vi "Create.vi"(8 "error in (no error)":errorcluster, 11 "DataSocketMessenger in":refnum<class "DataSocketMessenger.lvclass">) -> (0 "error out":errorcluster, 3 "DataSocketMessenger out":refnum<class "DataSocketMessenger.lvclass">)   [LabVIEW 2011, in "Messenging.lvlib" / "DataSocketMessenger.lvclass"]
uses:
  DataSocketMessenger.lvclass
  DataSocketMessenger.lvclass/DataSocketMessenger.ctl
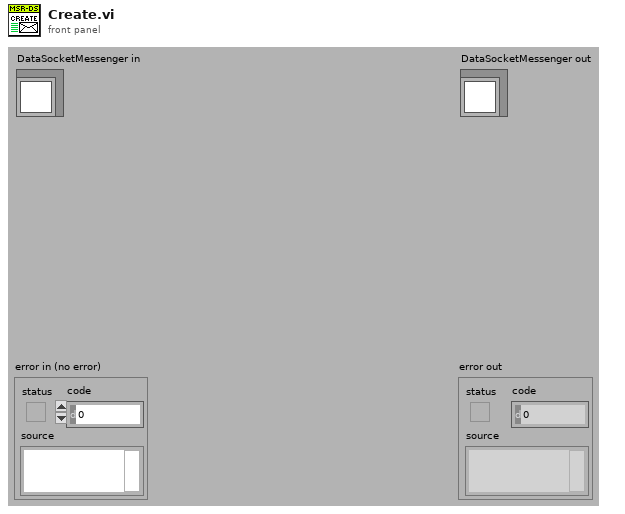
[diagram p1: front panel]
types:
  T1 = enum16{"Read", "Write", "ReadWrite", "BufferedRead", "BufferedReadWrite"}
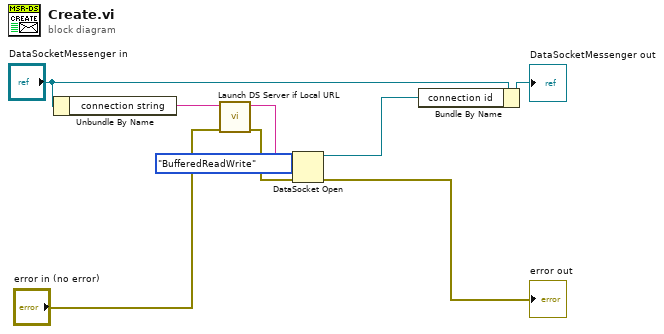
[diagram p0: block diagram]
diagram:
  n1 = Unbundle By Name("DataSocketMessenger in") -> ("connection string"=w9:string)
  n2 = call "Launch DS Server if Local URL.vi"("error in (no error)"="error in (no error)", "URL"=w9) -> ("error out"=w3:errorcluster, "Duplicate URL"=w8:string)  [unwired: 4 out]
  n3 = DataSocket Open(8:w3, 10:T1."BufferedReadWrite" ("mode"), 11:w8) -> (0:→"error out":errorcluster, 3:w5:refnum<k13>)  [unwired: 1 out]
  n4 = Bundle By Name(cluster="DataSocketMessenger in", "connection id"=w5) -> (→"DataSocketMessenger out":refnum<class "DataSocketMessenger.lvclass">)
